vi "Run Prompt with IMG.vi"(7 "Prompt text":string="What object do you see on the attached image.", 8 "error in (no error)":errorcluster, 10 "API key":string, 11 "path to JPEG file":path=path "C:/batt/IMG_3307.jpg") -> (0 "error out":errorcluster, 3 "body":string)   [LabVIEW 2025, in "Battery Prompt.lvlib"]
doc: "Executes a prompt that includes an image. Provide the prompt text, the path to the JPEG file and the API key for OpenAI."
uses:
  Battery Prompt.lvlib
  <vilib>/httpClient/POSTBuffer.vi
  <vilib>/httpClient/LabVIEWHTTPClient.lvlib
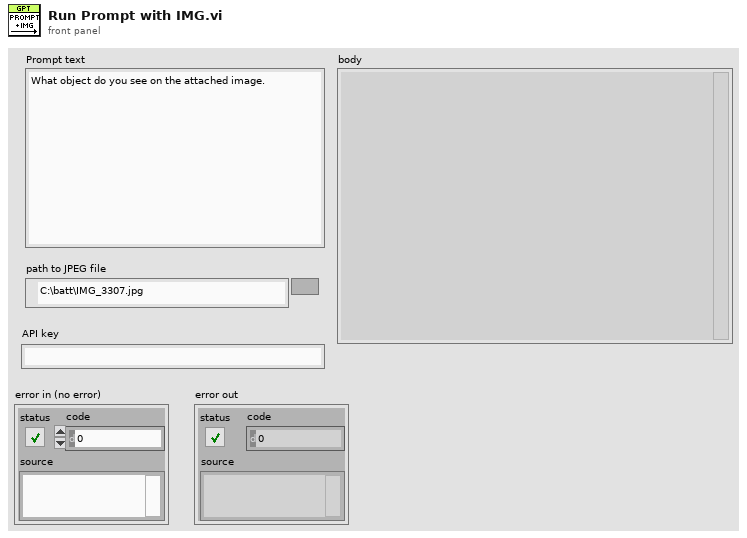
[diagram p1: front panel]
types:
  T1 = typedef "LabVIEWHTTPClient.lvlib/ClientHandle.ctl" = refnum<k1>
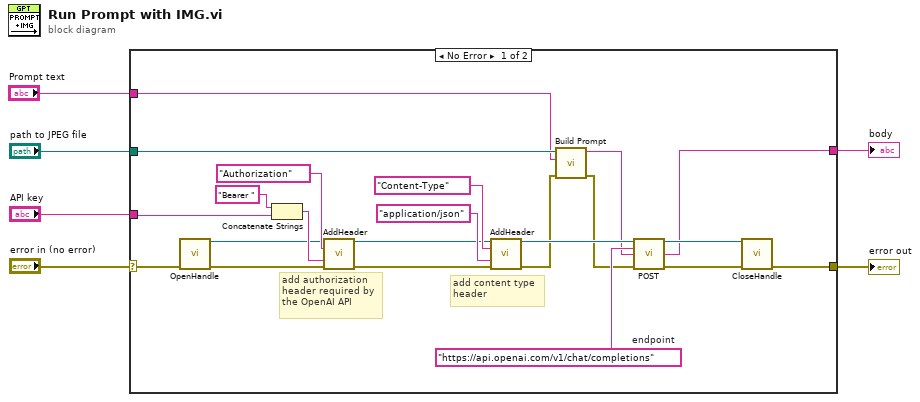
[diagram p0: block diagram]
diagram:
  n1 = case shown="No Error" "error in (no error)" {
    selector: "error in (no error)" -> [w17 w29]
    tunnel: [w13 w29] -> w5
    tunnel: "API key" -> [w18 _]
    tunnel: "path to JPEG file" -> [w12 _]
    tunnel: [w8 _] -> w2
    tunnel: "Prompt text" -> [w7 _]
    frame No Error {
      w28 = "https://api.openai.com/v1/chat/completions"  # endpoint
      # "add content type\nheader"
      # "add authorization\nheader required by\nthe OpenAI API"
      n2 = call <vilib>:"OpenHandle.vi"("error in (no error)"=w17) -> ("client handle out"=w20:T1, "error out"=w16:errorcluster)  [unwired: 13 in]
      n3 = Concatenate Strings("Bearer " ("string"), w18) -> (w21:string)
      n4 = call <vilib>:"AddHeader.vi"("client handle"=w20, "header"="Authorization", "value"=w21, "error in (no error)"=w16) -> ("client handle out"=w19:T1, "error out"=w15:errorcluster)  [unwired: 10 in]
      n5 = call <vilib>:"AddHeader.vi"("client handle"=w19, "header"="Content-Type", "value"="application/json", "error in (no error)"=w15) -> ("client handle out"=w25:T1, "error out"=w10:errorcluster)  [unwired: 10 in]
      n6 = call "Build Prompt.vi"("error in (no error)"=w10, "Prompt text"=w7, "path to JPEG file"=w12) -> ("error out"=w9:errorcluster, "Prompt"=w11:string)  [unwired: 7 in]
      n7 = call-poly <vilib>:"POST.vi"("client handle"=w25, "url"=w28, "buffer"=w11, "error in (no error)"=w9) -> ("client handle out"=w24:T1, "body"=w8:string, "error out"=w14:errorcluster)  [unwired: 8 in, 1 out]
      n8 = call <vilib>:"CloseHandle.vi"("client handle"=w24, "error in (no error)"=w14) -> ("error out"=w13:errorcluster)  [unwired: 13 in]
    }
    frame Error {
    }
  }
  "error out" <- w5
  "body" <- w2
